vi "Write MICROS.vi"(8 "error in (no error)":errorcluster, 10 "MICROS":T1, 11 "SERIAL DEVICE in":refnum<class "SERIAL DEVICE.lvclass">) -> (0 "error out":errorcluster, 3 "SERIAL DEVICE out":refnum<class "SERIAL DEVICE.lvclass">)   [LabVIEW 2019, in "SERIAL DEVICE.lvclass"]
uses:
  SERIAL DEVICE.lvclass
  MICROS.ctl
  SERIAL DEVICE.lvclass/SERIAL DEVICE.ctl
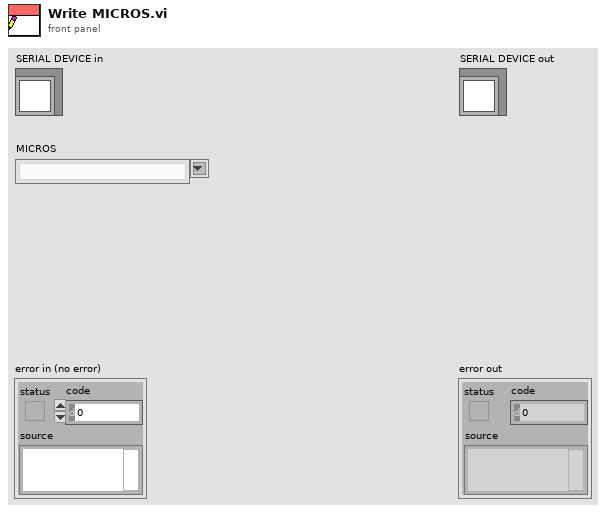
[diagram p1: front panel]
types:
  T1 = typedef "MICROS.ctl" = string
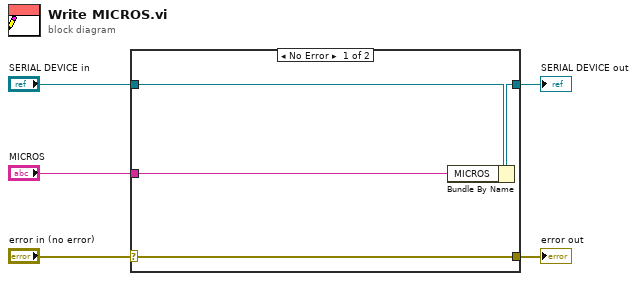
[diagram p0: block diagram]
diagram:
  n1 = case shown="No Error" "error in (no error)" {
    selector: "error in (no error)" -> [w9 w10]
    tunnel: [w9 w10] -> w4
    tunnel: [w7 w11] -> w2
    tunnel: "SERIAL DEVICE in" -> [w8 w11]
    tunnel: "MICROS" -> [w6 _]
    frame No Error {
      n2 = Bundle By Name(cluster=w8, "MICROS"=w6) -> (w7:refnum<class "SERIAL DEVICE.lvclass">)
    }
    frame Error {
    }
  }
  "error out" <- w4
  "SERIAL DEVICE out" <- w2
